vi "Cluster allarmi.vi"() -> ()   [LabVIEW 2016]
panel:
  out "Cluster ALARMS":T1
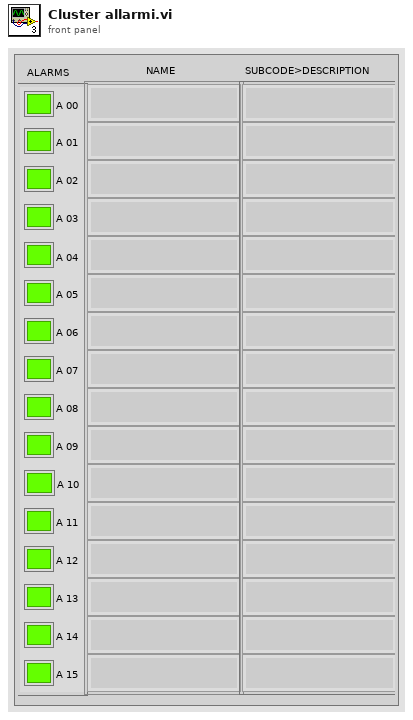
[diagram p1: front panel]
types:
  T1 = cluster{"ALARMS":cluster{"A 00":bool, "A 01":bool, "A 02":bool, "A 03":bool, "A 04":bool, "A 05":bool, "A 06":bool, "A 07":bool, "A 08":bool, "A 09":bool, "A 10":bool, "A 11":bool, "A 12":bool, "A 13":bool, "A 14":bool, "A 15":bool}, "DISABLE":cluster{"A 00":bool, "A 1":bool, "A 2":bool, "A 3":bool, "A 4":bool, "A 5":bool, "A 6":bool, "A 7":bool, "A 8":bool, "A 9":bool, "A 10":bool, "A 11":bool, "A 12":bool, "A 13":bool, "A 14":bool, "A 15":bool}, "NAME":string[], "SUBCODE>DESCRIPTION":string[]}
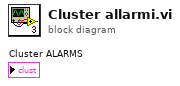
[diagram p0: block diagram]
diagram:
